vi "closeVIReferences.vi"(8 "error in (no error)":errorcluster, 11 "ProgrammaticInitialization in":refnum<class "ProgrammaticInitialization.lvclass">) -> (0 "error out":errorcluster, 3 "ProgrammaticInitialization out":refnum<class "ProgrammaticInitialization.lvclass">)   [LabVIEW 2016, in "ProgrammaticInitialization.lvclass"]
uses:
  ProgrammaticInitialization.lvclass
  ProgrammaticInitialization.lvclass/ProgrammaticInitialization.ctl
  <vilib>/Utility/Data Type/NI_Data Type.lvlib
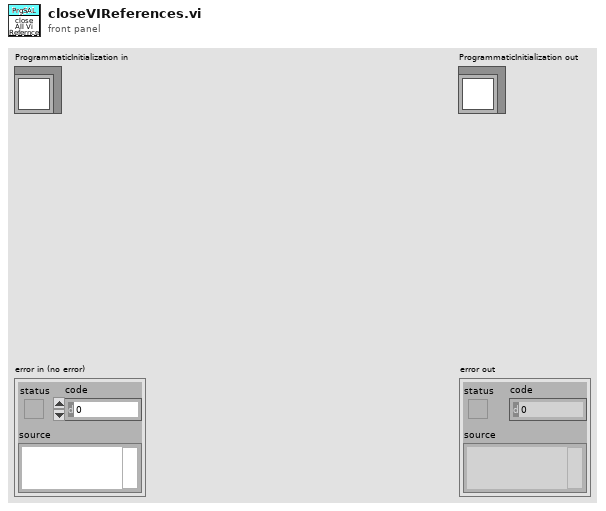
[diagram p1: front panel]
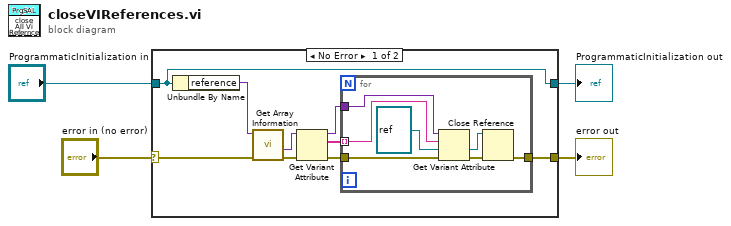
[diagram p0: block diagram]
diagram:
  n1 = case shown="No Error" "error in (no error)" {
    selector: "error in (no error)" -> [w10 w22]
    tunnel: [w7 w22] -> w3
    tunnel: [w13 w21] -> w1
    tunnel: "ProgrammaticInitialization in" -> [w13 w21]
    frame No Error {
      n2 = Unbundle By Name(w13) -> ("reference"=w12:variant)
      n3 = call <vilib>:"Get Array Information.vi"("error in (no error)"=w10, "Variant"=w12) -> ("error out"=w9:errorcluster, "Array Element Data Type"=w11:variant)  [unwired: 6 in, 2 out]
      n4 = Get Variant Attribute(Variant=w11, error in=w9) -> (duplicate Variant=w5:variant, names=w6:string[], error out=w8:errorcluster)  [unwired: 2 in, 1 out]
      n5 = for {
        tunnel: w8 -> [w19]
        tunnel: [w20] -> w7
        tunnel: w6 -> [w17] mode=indexing
        tunnel: w5 -> [w14]
        n6 = Get Variant Attribute(Variant=w14, name=w17, default value (empty Variant)=refnum<vi> refnum ("reference"), error in=w19) -> (value=w15:refnum<vi>, error out=w18:errorcluster)  [unwired: 2 out]
        n7 = Close Reference(reference=w15, error in (no error)=w18) -> (error out=w20:errorcluster)
      }
    }
    frame Error {
    }
  }
  "error out" <- w3
  "ProgrammaticInitialization out" <- w1
